vi "BC Verify Message Data.vi"(5 "Instruction ID":i32, 6 "Data Address":u16 format="%04x", 7 "Target IC (1-8)":u8, 8 "error in (no error)":errorcluster, 10 "RT-RT?":bool, 11 "Bus Controller in":refnum<class "Bus Controller.lvclass">) -> (0 "error out":errorcluster, 3 "Bus Controller out":refnum<class "Bus Controller.lvclass">, 4 "Post-Data Address":u16 format="%04x")   [LabVIEW 2020, in "Unit Tests.lvlib" / "Bus Controller.lvclass"]
uses:
  Bus Controller.lvclass
  Bus Controller.lvclass/Bus Controller.ctl
  <vilib>/addons/_JKI Toolkits/Caraya/classes/Assert/Assert True.vi
  Dependencies/FPGA Interface/FPGA Interface.lvclass
  <vilib>/addons/_JKI Toolkits/Caraya/classes/Test/Test.lvclass
  BCI-1553 API.lvlib
  <vilib>/addons/_JKI Toolkits/Caraya/classes/Assert/Assert.lvclass
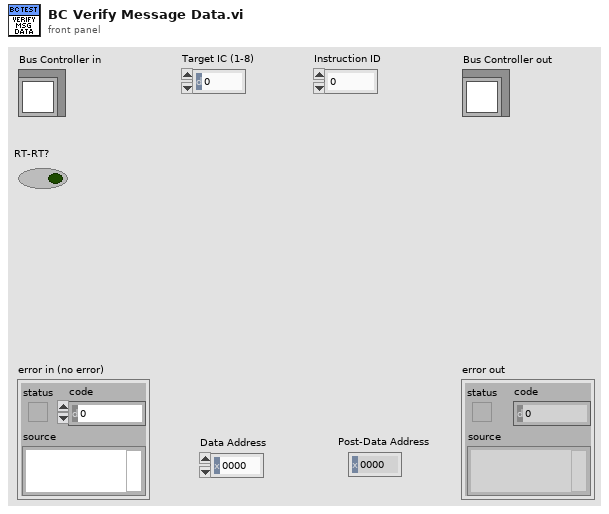
[diagram p1: front panel]
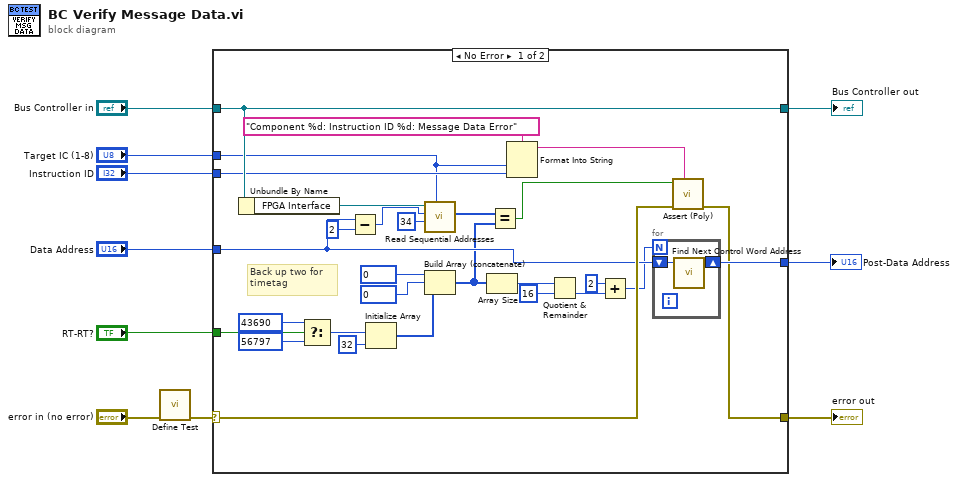
[diagram p0: block diagram]
diagram:
  n1 = call <vilib>:"Define Test.vi"("error in (no error)"="error in (no error)") -> ("error out"=w6:errorcluster)  [unwired: 9 in, 1 out]
  n2 = case shown="No Error" w6 {
    selector: w6 -> [w21 w44]
    tunnel: [w20 w44] -> w10
    tunnel: [w39 w43] -> w8
    tunnel: "Bus Controller in" -> [w39 w43]
    tunnel: "RT-RT?" -> [w31 _]
    tunnel: "Data Address" -> [w19 w42]
    tunnel: "Target IC (1-8)" -> [w26 _]
    tunnel: "Instruction ID" -> [w27 _]
    tunnel: [w24 w42] -> w1
    frame No Error {
      # "Back up two for \ntimetag"
      n3 = Unbundle By Name(w39) -> ("FPGA Interface"=w30:refnum<class "FPGA Interface.lvclass">)
      n4 = Select(t=u16 43690, s=w31, f=u16 56797) -> (s? t:f=w34:u16)
      n5 = Subtract(x=w19, y=u16 2) -> (x-y=w17:u16)
      n6 = Initialize Array(w34, 32 ("dimension size")) -> (w32:u16[])
      n7 = call-dynamic "Read Sequential Addresses.vi"("Target IC (1-8)"=w26, "Addresses to Read"=u16 34, "Starting Address"=w17, "FPGA Interface in"=w30) -> ("Data"=w25:u16[])  [unwired: 6 in, 1 out]
      n8 = Build Array (concatenate)(u16 0, u16 0, w32) -> (w12:u16[])
      n9 = Array Size(array=w12) -> (size(s)=w16:i32)
      n10 = Equal?(x=w25, y=w12) -> (x = y?=w23:bool)
      n11 = Format Into String(format string="Component %d: Instruction ID %d: Message Data Error" ("message (\"\")"), w26, w27) -> (resulting string=w22:string)  [unwired: 2 in, 1 out]
      n12 = Quotient & Remainder(x=w16, y=16) -> (floor(x/y)=w14:i32)  [unwired: 1 out]
      n13 = Add(x=2, y=w14) -> (x+y=w11:i32)
      n14 = for {
        N: w11 -> [_]
        shift-right: [w40] -> w24
        shift-left: w19 -> [w41]
        n15 = call "Find Next Control Word Address.vi"("Starting Address"=w41) -> ("0xHHHX Address"=w40:u16)  [unwired: 10 in]
      }
      n16 = call-poly <vilib>:"Assert (Poly).vi"("Label"=w22, "error in (no error)"=w21, "True?"=w23) -> ("error out"=w20:errorcluster)  [unwired: 7 in, 1 out]
    }
    frame Error {
    }
  }
  "error out" <- w10
  "Bus Controller out" <- w8
  "Post-Data Address" <- w1
